vi "View Log.vi"(8 "error in (no error)":errorcluster, 11 "Rename in":refnum<class "Rename.lvclass">) -> (0 "error out":errorcluster, 3 "Rename out":refnum<class "Rename.lvclass">)   [LabVIEW 2015, in "Generic Module Library.lvlib" / "Template G_Module.lvlib" / "Rename.lvclass"]
uses:
  Rename.lvclass
  Template G_Module.lvlib
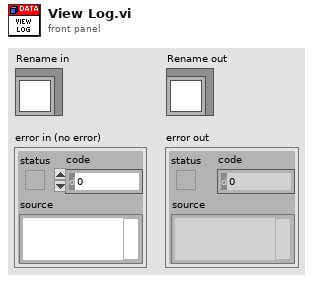
[diagram p1: front panel]
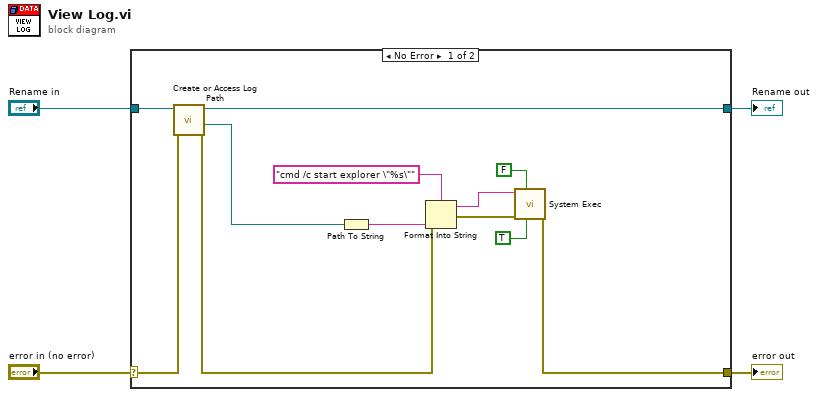
[diagram p0: block diagram]
diagram:
  n1 = case shown="No Error" "error in (no error)" {
    selector: "error in (no error)" -> [w14 w18]
    tunnel: [w10 w18] -> w3
    tunnel: [w15 w17] -> w1
    tunnel: "Rename in" -> [w16 w17]
    frame No Error {
      n2 = call "Create or Access Log Path.vi"("error in"=w14, "Module Data In"=w16) -> ("error out"=w6:errorcluster, "Log Path"=w13:path, "Module Data Out"=w15:refnum<class "Rename.lvclass">)  [unwired: 6 in, 1 out]
      n3 = Path To String(path=w13) -> (string=w7:string)
      n4 = Format Into String(format string="cmd /c start explorer \"%s\"", error in=w6, w7) -> (resulting string=w11:string, error out=w5:errorcluster)  [unwired: 1 in]
      n5 = call <vilib>:"System Exec.vi"("run minimized? (F)"=TRUE, "wait until completion? (T)"=FALSE, "error in (no error)"=w5, "command line"=w11) -> ("error out"=w10:errorcluster)  [unwired: 4 in, 3 out]
    }
    frame Error {
    }
  }
  "error out" <- w3
  "Rename out" <- w1
